vi "dataCollection.vi"() -> ()   [LabVIEW 2017]
panel:
  in  "COM port":refnum<visa-resource-name>="COM1"
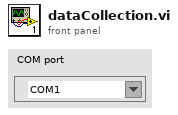
[diagram p1: front panel]
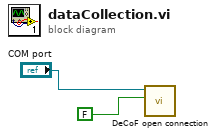
[diagram p0: block diagram]
diagram:
  n1 = call "DeCoF open connection.vi"("TCP?"=FALSE, "address"="COM port") -> ()  [unwired: 4 in, 2 out]
